vi "Read PmuDataArray.vi"(8 "error in (no error)":errorcluster, 11 "PmuBase in":refnum<class "PmuBase.lvclass">) -> (0 "error out":errorcluster, 2 "PmuDataArray":T1[](array[typedef]) {"Synx" format="%#_4g"}, 3 "PmuBase out":refnum<class "PmuBase.lvclass">)   [LabVIEW 2014, in "SensorPlugins.lvlib" / "PmuBase.lvclass"]
uses:
  PmuBase.lvclass
  Typedef/PmuData.ctl
  PmuBase.lvclass/PmuBase.ctl
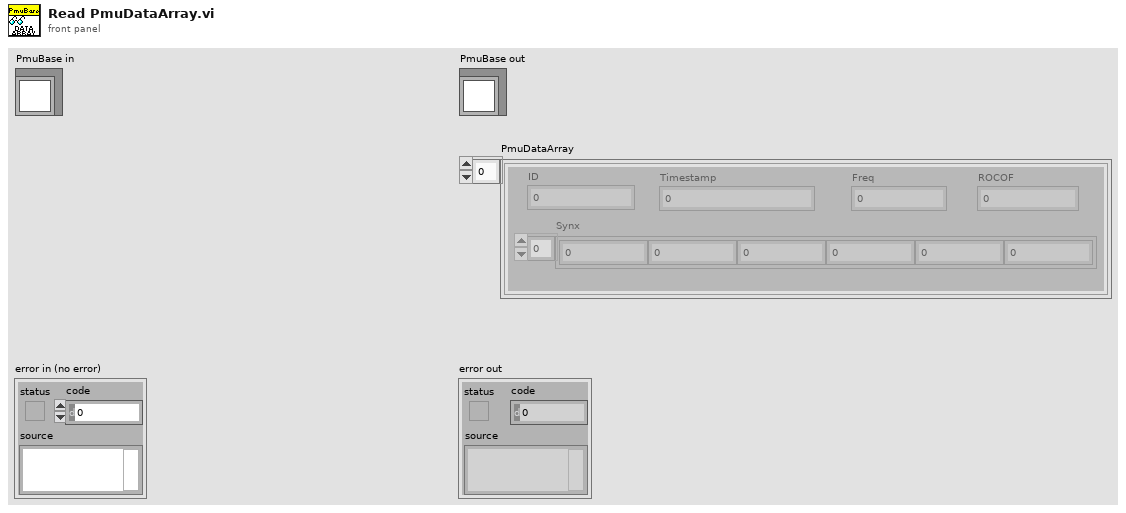
[diagram p1: front panel]
types:
  T1 = typedef "SensorPlugins.lvlib/PmuBase.lvclass/PmuData.ctl" = cluster{"Timestamp":dbl, "Synx":cdb[], "Freq":dbl, "ROCOF":dbl, "ID":i16}
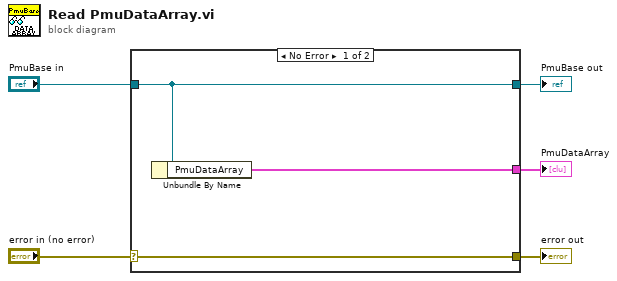
[diagram p0: block diagram]
diagram:
  n1 = case shown="No Error" "error in (no error)" {
    selector: "error in (no error)" -> [w8 w9]
    tunnel: [w8 w9] -> w4
    tunnel: [w7 w10] -> w2
    tunnel: "PmuBase in" -> [w7 w10]
    tunnel: [w6 _] -> w1
    frame No Error {
      n2 = Unbundle By Name(w7) -> ("PmuDataArray"=w6:T1[])
    }
    frame Error {
    }
  }
  "error out" <- w4
  "PmuBase out" <- w2
  "PmuDataArray" <- w1
